vi "hwave.vi"() -> ()   [LabVIEW 2023]
panel:
  out "Waveform Chart":dbl(graph)
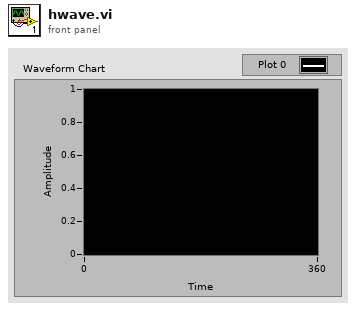
[diagram p1: front panel]
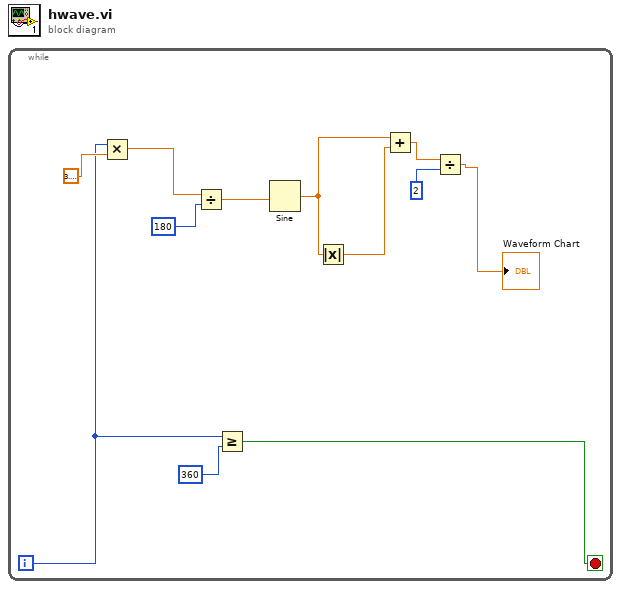
[diagram p0: block diagram]
diagram:
  n1 = while {
    i -> [w6]
    stop <- w4 stop-if-true
    n2 = Multiply(x=w6, y=3.141592653589793) -> (x*y=w11:dbl)
    n3 = Divide(x=w11, y=180) -> (x/y=w9:dbl)
    n4 = Greater Or Equal?(x=w6, y=360) -> (x >= y?=w4:bool)
    n5 = Sine(x=w9) -> (sin(x)=w8:dbl)
    n6 = Absolute Value(x=w8) -> (abs(x)=w7:dbl)
    n7 = Add(x=w8, y=w7) -> (x+y=w2:dbl)
    n8 = Divide(x=w2, y=2) -> (x/y=→"Waveform Chart":dbl)
  }
